vi "RomiGyro_PanelSim_Global.vi"(0 "Menu":T3=enum."delete", 5 "Channel":i32, 7 "Boolean Value":bool, 9 "Numeric Value":dbl format="%#.4f", 11 "error in (no error)":errorcluster, 12 "String Value":string) -> (10 "Value out":T1={"type"="AI", "device"="", "name"="", "data"={"<init"=0, ">connected"=FALSE, "<offsetX"=0.0, "<offsetY"=0.0, "<offsetZ"=0.0, ">angle_x"=0.0, ">angle_y"=0.0, ">angle_z"=0.0, ">rate_x"=0.0, ">rate_y"=0.0, ">rate_z"=0.0, "<gain"=0.0}}, 15 "error out":errorcluster)   [LabVIEW 2019]
doc: "This is used to set and get the last motor output values. This is needed for simulation, since we cannot read these values from the hardware.\n\nThis software is licensed. Open the labview\\readme\\WPI Robotics Library Open Source License.txt file for more information."
uses:
  RomiGyro Data proto.ctl
  RomiGyro proto.ctl
  RomiGyro Update Ops.ctl
panel:
  out "All Values":T1[](array[typedef])
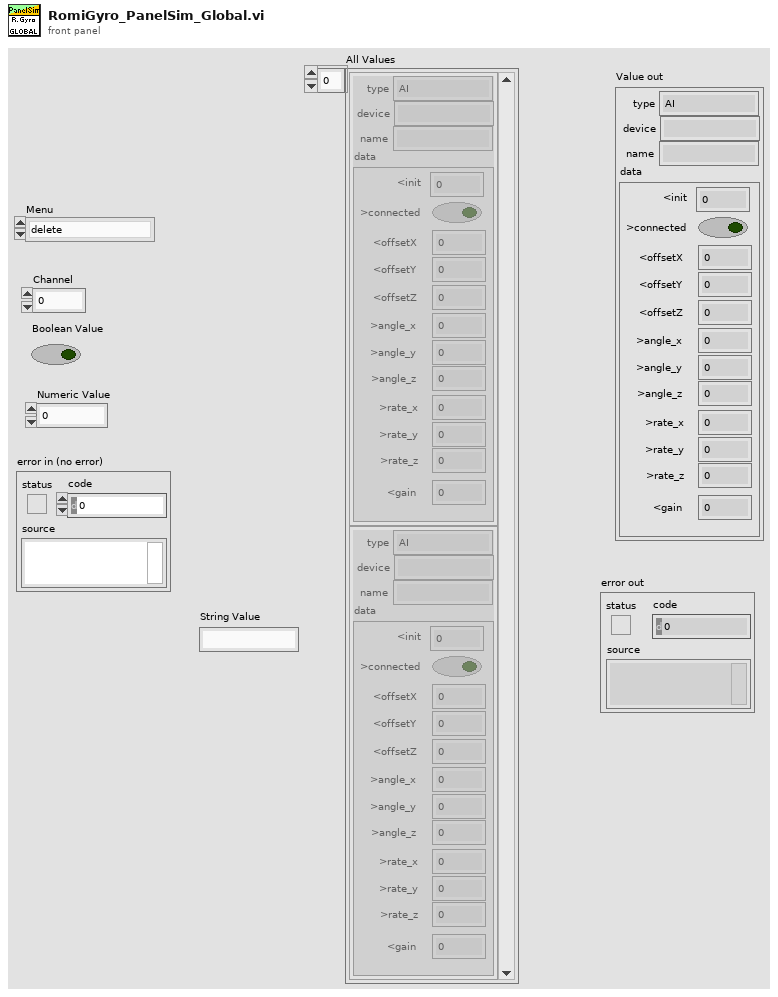
[diagram p1: front panel]
types:
  T1 = typedef "RomiGyro proto.ctl" = cluster{"type":string, "device":string, "name":string, "data":T2}
  T2 = typedef "RomiGyro Data proto.ctl" = cluster{"<init":i32, ">connected":bool, "<offsetX":dbl, "<offsetY":dbl, "<offsetZ":dbl, ">angle_x":dbl, ">angle_y":dbl, ">angle_z":dbl, ">rate_x":dbl, ">rate_y":dbl, ">rate_z":dbl, "<gain":dbl}
  T3 = typedef "RomiGyro Update Ops.ctl" = enum16{"get", "delete", "JSON update", "set  name", "transmit initial", "reset", "set init", "set offsetX", "set offsetY", "set offsetZ", "set gain", "set angle X", "set angle Y", "set angle Z", "set rate X", "set rate Y", "set rate Z"}
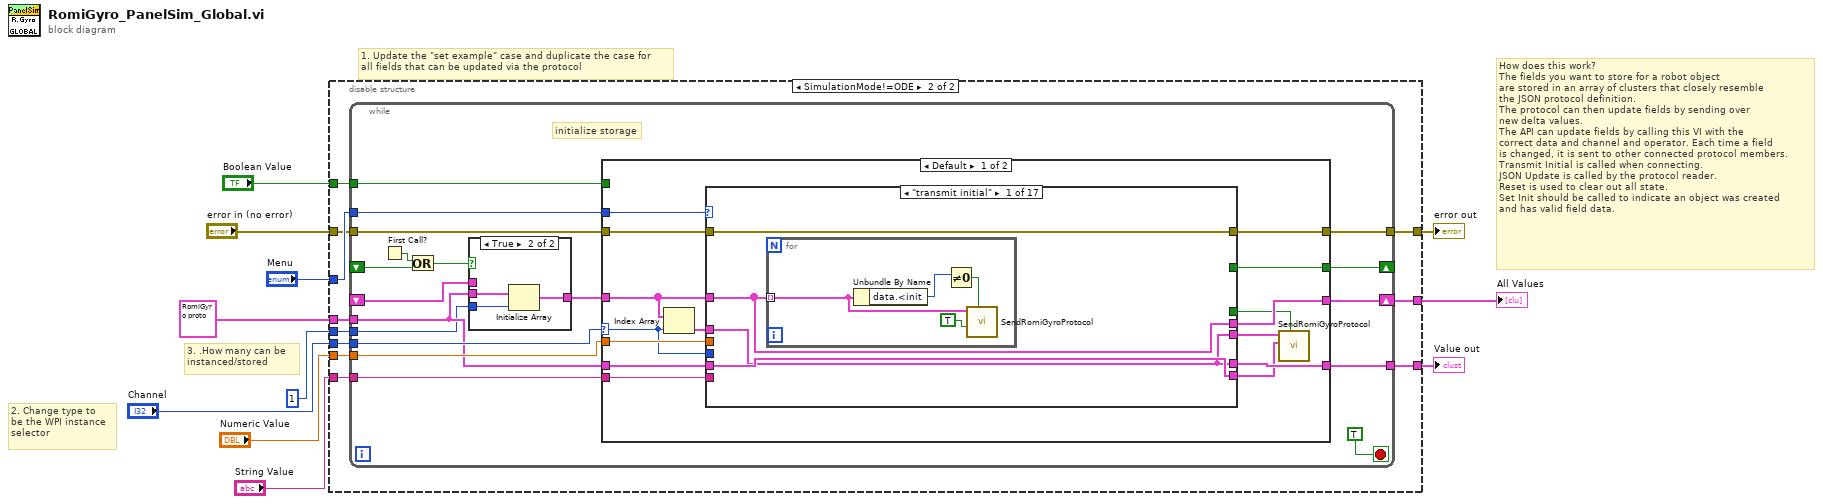
[diagram p0: block diagram]
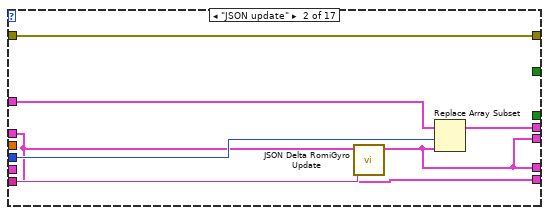
[diagram p3: hidden frame]
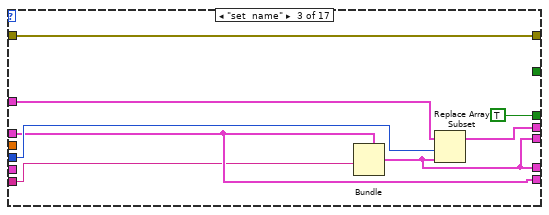
[diagram p4: hidden frame]
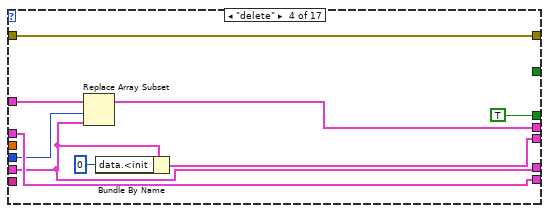
[diagram p5: hidden frame]
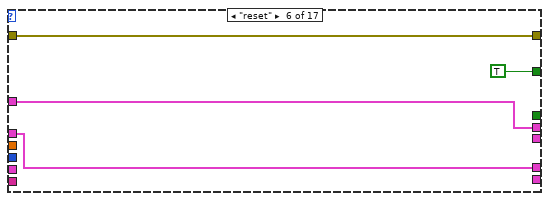
[diagram p7: hidden frame]
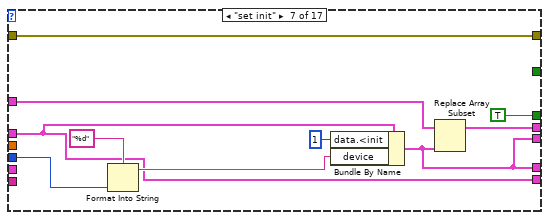
[diagram p8: hidden frame]
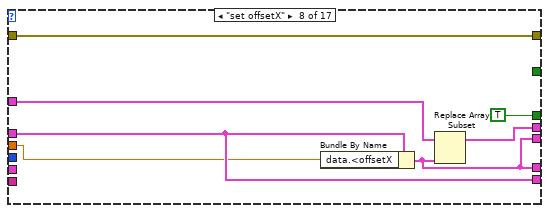
[diagram p9: hidden frame]
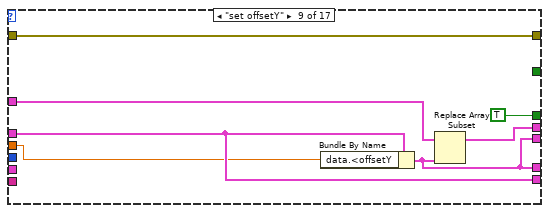
[diagram p10: hidden frame]
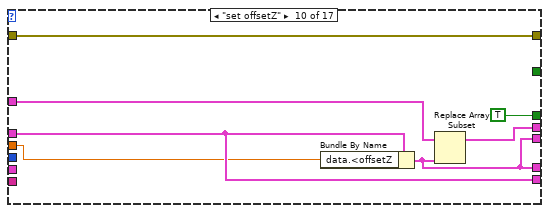
[diagram p11: hidden frame]
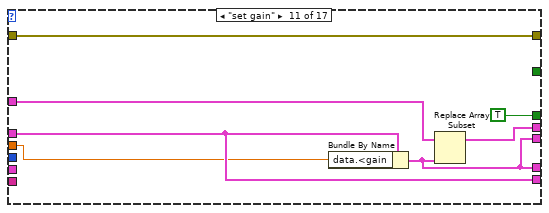
[diagram p12: hidden frame]
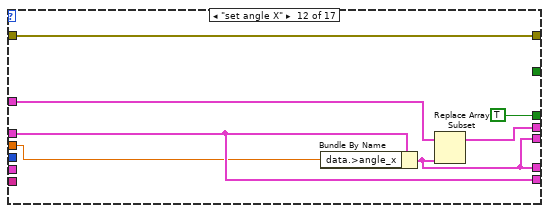
[diagram p13: hidden frame]
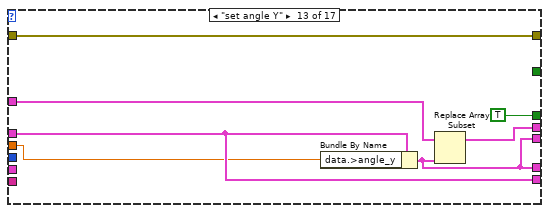
[diagram p14: hidden frame]
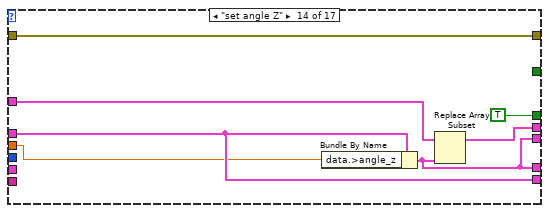
[diagram p15: hidden frame]
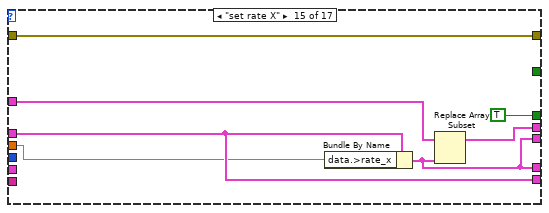
[diagram p16: hidden frame]
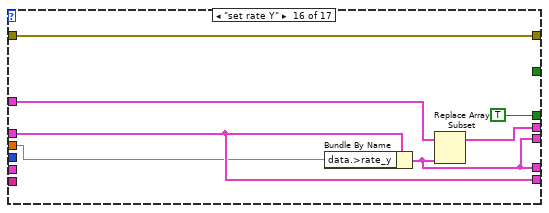
[diagram p17: hidden frame]
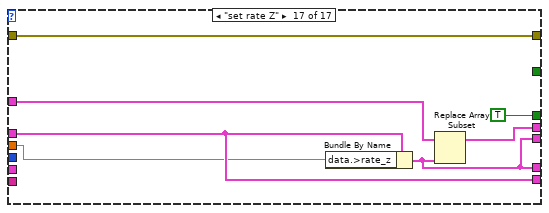
[diagram p18: hidden frame]
diagram:
  # "How does this work?\nThe fields you want to store for a robot object\nare stored in an array of clusters that closely resemble\nthe JSON protocol definition.\nThe protocol can then update fields by sending over\nnew delta values.\nThe API can update fields by calling this VI with the\ncorrect data and channel and operator. Each time a field\nis changed, it is sent to other connected protocol members.\nTransmit Initial is called when connecting.\nJSON Update is called by the protocol reader.\nReset is used to clear out all state.\nSet Init should be called to indicate an object was created\nand has valid field data."
  # "1. Update the \"set example\" case and duplicate the case for\nall fields that can be updated via the protocol"
  # "2. Change type to\nbe the WPI instance\nselector"
  # "3. .How many can be\ninstanced/stored"
  n1 = disable-structure shown="SimulationMode!=ODE" {
    disable-tunnel: "Menu" -> [_ w24]
    disable-tunnel: [w13 w23] -> w10
    disable-tunnel: "error in (no error)" -> [w13 w22]
    disable-tunnel: [_ w21] -> w8
    disable-tunnel: "Numeric Value" -> [_ w20]
    disable-tunnel: "Channel" -> [_ w19]
    disable-tunnel: [w12 w18] -> w5
    disable-tunnel: T1 {"type"="Gyro", "device"="", "name"="", "data"={"<init"=0, ">connected"=FALSE, "<offsetX"=0.0, "<offsetY"=0.0, "<offsetZ"=0.0, ">angle_x"=0.0, ">angle_y"=0.0, ">angle_z"=0.0, ">rate_x"=0.0, ">rate_y"=0.0, ">rate_z"=0.0, "<gain"=0.0}} ("Accel value out") -> [w12 w17]
    disable-tunnel: "String Value" -> [_ w16]
    disable-tunnel: 1 -> [_ w15]
    disable-tunnel: "Boolean Value" -> [_ w14]
    frame condition #0 {
    }
    frame condition #1 (active) {
      n2 = while {
        tunnel: w20 -> [w42]
        tunnel: w22 -> [w38]
        shift-right: [w41] -> w21
        shift-left: _ -> [w34]
        tunnel: [w40] -> w18
        tunnel: w24 -> [w39]
        tunnel: [w37] -> w23
        tunnel: w19 -> [w33]
        tunnel: w17 -> [w32]
        tunnel: w16 -> [w31]
        shift-right: [w27] -> _
        shift-left: _ -> [w28]
        tunnel: w15 -> [w26]
        tunnel: w14 -> [w25]
        stop <- TRUE stop-if-true
        # "initialize storage"
        n3 = First Call?() -> (First Call?: T/F=w29:bool)
        n4 = Or(x=w29, y=w28) -> (x .or. y?=w30:bool)
        n5 = case shown="True" w30 {
          tunnel: [w180 w183] -> w35
          tunnel: w34 -> [w180 _]
          tunnel: w32 -> [_ w182]
          tunnel: w26 -> [_ w181]
          frame False {
          }
          frame True {
            n6 = Initialize Array(w182, w181) -> (w183:T1[])
          }
        }
        n7 = case shown="Default" w33 {
          selector: w33 -> [w50 _]
          tunnel: w42 -> [w57 _]
          tunnel: [w56 w179] -> w41
          tunnel: [w55 w177] -> w40
          tunnel: w39 -> [w54 _]
          tunnel: w38 -> [w53 w178]
          tunnel: [w52 w178] -> w37
          tunnel: w35 -> [w51 w179]
          tunnel: w32 -> [w48 w177]
          tunnel: w31 -> [w47 _]
          tunnel: [w46 _] -> w27
          tunnel: w25 -> [_ _]
          frame Default {
            n8 = Index Array(array=w51, index=w50) -> (element=w49:T1)
            n9 = case shown="\"transmit initial\"" w54 {
              tunnel: w57 -> [_ _ _ _ _ _ _ w107 w114 w121 w128 w135 w142 w149 w156 w163 w170]
              tunnel: [w58 w72 w80 w88 w92 w96 w102 w112 w119 w126 w133 w140 w147 w154 w161 w168 w175] -> w56
              tunnel: w51 -> [w58 w70 w78 w89 w92 w96 w101 w111 w118 w125 w132 w139 w146 w153 w160 w167 w174]
              tunnel: [w59 w68 w73 w82 w90 w94 w99 w109 w116 w123 w130 w137 w144 w151 w158 w165 w172] -> w55
              tunnel: [w61 w71 w79 w87 w91 w95 w98 w108 w115 w122 w129 w136 w143 w150 w157 w164 w171] -> w52
              tunnel: w53 -> [w61 w71 w79 w87 w91 w95 w98 w108 w115 w122 w129 w136 w143 w150 w157 w164 w171]
              tunnel: w50 -> [_ w69 w76 w84 _ _ w105 _ _ _ _ _ _ _ _ _ _]
              tunnel: [w59 w68 w73 w83 _ _ w99 w109 w116 w123 w130 w137 w144 w151 w158 w165 w172] -> w44
              tunnel: [w60 w66 w75 w85 _ _ w100 w110 w117 w124 w131 w138 w145 w152 w159 w166 w173] -> w43
              tunnel: [_ _ TRUE TRUE _ _ TRUE TRUE TRUE TRUE TRUE TRUE TRUE TRUE TRUE TRUE TRUE] -> w45
              tunnel: w49 -> [w59 w66 w75 w85 w90 w94 w100 w110 w117 w124 w131 w138 w145 w152 w159 w166 w173]
              tunnel: w48 -> [w60 _ _ w82 _ _ _ _ _ _ _ _ _ _ _ _ _]
              tunnel: w47 -> [_ w67 w74 _ _ _ _ _ _ _ _ _ _ _ _ _ _]
              tunnel: [_ _ _ _ _ TRUE _ _ _ _ _ _ _ _ _ _ _] -> w46
              frame "transmit initial" {
                n10 = for {
                  tunnel: w58 -> [w65] mode=indexing
                  n11 = Unbundle By Name(w65) -> ("data.<init"=w62:i32)
                  n12 = Not Equal To 0?(x=w62) -> (x != 0?=w63:bool)
                  n13 = call "SendRomiGyroProtocol.vi"("Send"=w63, "Initialize"=TRUE ("Send"), "Current"=w65) -> ()  [unwired: 9 in]
                }
              }
              frame "JSON update" {
                n14 = call "JSON Delta RomiGyro Update.vi"("Delta JSON"=w67, "input"=w66) -> ("output"=w68:T1)  [unwired: 8 in, 1 out]
                n15 = Replace Array Subset(array=w70, new element=w68, index=w69) -> (w72:T1[])
              }
              frame "set  name" {
                n16 = Bundle(cluster=w75, "name"=w74) -> (w73:T1)  [unwired: 3 in]
                n17 = Replace Array Subset(array=w78, new element=w73, index=w76) -> (w80:T1[])
              }
              frame "delete" {
                n18 = Replace Array Subset(array=w89, new element=w82, index=w84) -> (w88:T1[])
                n19 = Bundle By Name(cluster=w82, "data.<init"=0) -> (w83:T1)
              }
              frame "get" {
              }
              frame "reset" {
              }
              frame "set init" {
                n20 = Format Into String(format string="%d", w105) -> (resulting string=w104:string)  [unwired: 2 in, 1 out]
                n21 = Bundle By Name(cluster=w100, "data.<init"=1, "device"=w104) -> (w99:T1)
                n22 = Replace Array Subset(array=w101, new element=w99) -> (w102:T1[])  [unwired: 1 in]
              }
              frame "set offsetX" {
                n23 = Bundle By Name(cluster=w110, "data.<offsetX"=w107) -> (w109:T1)
                n24 = Replace Array Subset(array=w111, new element=w109) -> (w112:T1[])  [unwired: 1 in]
              }
              frame "set offsetY" {
                n25 = Bundle By Name(cluster=w117, "data.<offsetY"=w114) -> (w116:T1)
                n26 = Replace Array Subset(array=w118, new element=w116) -> (w119:T1[])  [unwired: 1 in]
              }
              frame "set offsetZ" {
                n27 = Bundle By Name(cluster=w124, "data.<offsetZ"=w121) -> (w123:T1)
                n28 = Replace Array Subset(array=w125, new element=w123) -> (w126:T1[])  [unwired: 1 in]
              }
              frame "set gain" {
                n29 = Bundle By Name(cluster=w131, "data.<gain"=w128) -> (w130:T1)
                n30 = Replace Array Subset(array=w132, new element=w130) -> (w133:T1[])  [unwired: 1 in]
              }
              frame "set angle X" {
                n31 = Bundle By Name(cluster=w138, "data.>angle_x"=w135) -> (w137:T1)
                n32 = Replace Array Subset(array=w139, new element=w137) -> (w140:T1[])  [unwired: 1 in]
              }
              frame "set angle Y" {
                n33 = Bundle By Name(cluster=w145, "data.>angle_y"=w142) -> (w144:T1)
                n34 = Replace Array Subset(array=w146, new element=w144) -> (w147:T1[])  [unwired: 1 in]
              }
              frame "set angle Z" {
                n35 = Bundle By Name(cluster=w152, "data.>angle_z"=w149) -> (w151:T1)
                n36 = Replace Array Subset(array=w153, new element=w151) -> (w154:T1[])  [unwired: 1 in]
              }
              frame "set rate X" {
                n37 = Bundle By Name(cluster=w159, "data.>rate_x"=w156) -> (w158:T1)
                n38 = Replace Array Subset(array=w160, new element=w158) -> (w161:T1[])  [unwired: 1 in]
              }
              frame "set rate Y" {
                n39 = Bundle By Name(cluster=w166, "data.>rate_y"=w163) -> (w165:T1)
                n40 = Replace Array Subset(array=w167, new element=w165) -> (w168:T1[])  [unwired: 1 in]
              }
              frame "set rate Z" {
                n41 = Bundle By Name(cluster=w173, "data.>rate_z"=w170) -> (w172:T1)
                n42 = Replace Array Subset(array=w174, new element=w172) -> (w175:T1[])  [unwired: 1 in]
              }
            }
            n43 = call "SendRomiGyroProtocol.vi"("Send"=w45, "Previous"=w43, "Current"=w44) -> ()  [unwired: 9 in]
          }
          frame -1 {
            # "Do nothing if \nchannel is Invalid."
          }
        }
      }
    }
  }
  "error out" <- w10
  "Value out" <- w5
  "All Values" <- w8
